vi "Set grid parameters (SubVI).vi"() -> (0 "number of spots":i32, 1 "Z":sgl[](array[numeric]), 2 "Y":sgl[](array[numeric]), 3 "X":sgl[](array[numeric]), 4 "I":sgl[](array[numeric]))   [LabVIEW 2011]
panel:
  in  "Offset y":sgl
  in  "Offset x":sgl
  in  "stop":bool
  in  "I":sgl=1.0
  in  "Z":sgl
  in  "Grid spacing":sgl
  in  "Spots y":i32
  in  "Spots x":i32
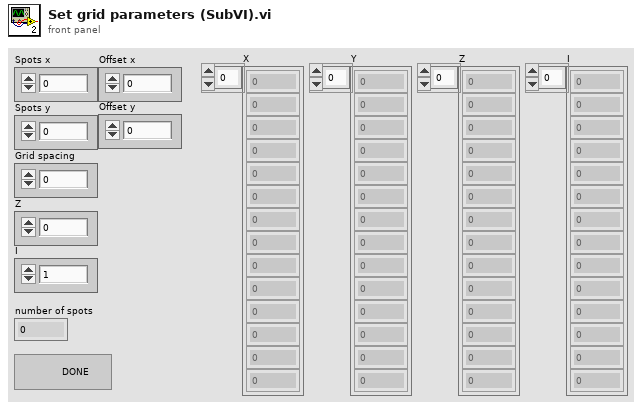
[diagram p1: front panel]
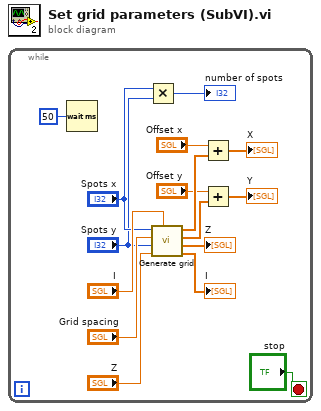
[diagram p0: block diagram]
diagram:
  n1 = while {
    stop <- "stop" stop-if-true
    n2 = Wait (ms)(milliseconds to wait=u32 50) -> ()  [unwired: 1 out]
    n3 = Multiply(x="Spots x", y="Spots y") -> (x*y=→"number of spots":i32)
    n4 = call "Generate grid.vi"("I"="I", "Z"="Z", "Spots y"="Spots y", "Grid spacing"="Grid spacing", "Spots x"="Spots x") -> ("I"=→"I":sgl[], "Z"=→"Z":sgl[], "Y"=w4:sgl[], "X"=w5:sgl[])
    n5 = Add(x="Offset x", y=w5) -> (x+y=→"X":sgl[])
    n6 = Add(x="Offset y", y=w4) -> (x+y=→"Y":sgl[])
  }
